vi "Main.vi"(8 "Error In":errorcluster, 10 "Output Root Directory":path=path "C:/Users/samkristoff/Desktop/dokugen output") -> (0 "Error Out":errorcluster)   [LabVIEW 2014]
panel:
  in  "Common Related Link(s)":string="[[learn:libraries:linx:reference:labview:start]] \\\\"
  in  "Relative Wiki Path":string="learn:libraries:linx:reference:labview:"
  in  "Wik Help Base URL":string="https://www.labviewmakerhub.com/doku.php?id=learn:libraries:linx:reference:labview:"
  in  "Folder Path":path=path "C:/github/makerhub/LINX/LabVIEW/vi.lib/MakerHub/LINX/Public"
  out "Progress":u8(slide)=99 scale=0.0..100.0
  out "File Path Control":path=path "C:/Program Files (x86)/National Instruments/LabVIEW 2014/vi.lib/MakerHub/LINX/Public/Utilities/Set Device User ID.vi"
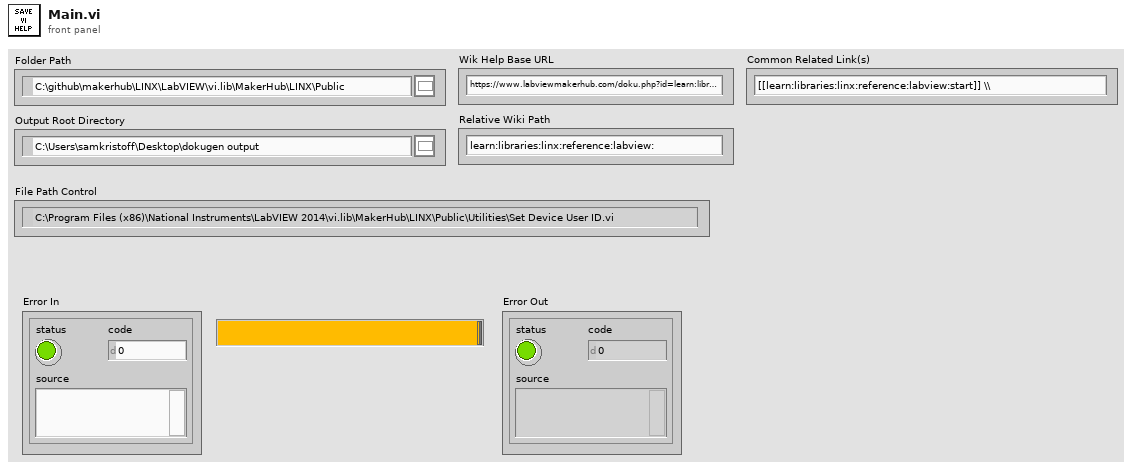
[diagram p1: front panel]
types:
  T1 = typedef "VI Data.ctl" = cluster{"Name":string, "Description":string, "Controls":T2[], "Indicators":T2[], "Connector Pane Image Data":T3, "Block Diagram Image Data":T3, "Path Tokens":string[]}
  T2 = typedef "Control Info.ctl" = cluster{"Label":string, "Description":string}
  T3 = typedef "imagedata.ctl" = cluster{"image type":i32, "image depth":i32, "image":u8[], "mask":u8[], "colors":u32[], "Rectangle":cluster{"left":i16, "top":i16, "right":i16, "bottom":i16}}
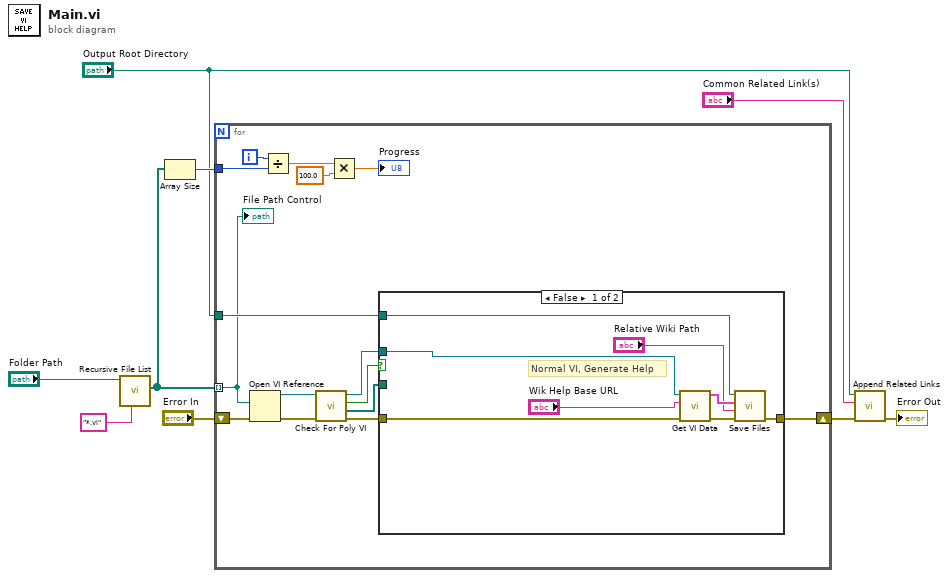
[diagram p0: block diagram]
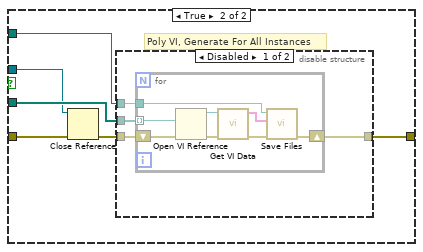
[diagram p2: hidden frame]
diagram:
  n1 = call <vilib>:"Recursive File List.vi"("pattern"="*.vi", "Folder Path"="Folder Path") -> ("All Files in Dir"=w6:path[])  [unwired: 5 in, 4 out]
  n2 = Array Size(array=w6) -> (size(s)=w5:i32)
  n3 = for {
    tunnel: "Output Root Directory" -> [w21]
    shift-right: [w20] -> w2
    shift-left: "Error In" -> [w17]
    tunnel: w6 -> [w16] mode=indexing
    tunnel: w5 -> [w13]
    i -> [w14]
    n4 = Open VI Reference(vi path=w16, error in (no error)=w17) -> (vi reference=w15:refnum<vi>, error out=w18:errorcluster)  [unwired: 4 in]
    n5 = Divide(x=w14, y=w13) -> (x/y=w12:dbl)
    n6 = call "Check For Poly VI.vi"("Error In"=w18, "VI Reference"=w15) -> ("Error Out"=w22:errorcluster, "Dependency Paths"=w23:path[], "Poly VI?"=w24:bool, "VI Reference"=w19:refnum<vi>)  [unwired: 6 in]
    n7 = Multiply(x=w12, y=100.0) -> (x*y=→"Progress":dbl)
    n8 = case shown="False" w24 {
      tunnel: w23 -> [_ w38]
      tunnel: w22 -> [w31 w34]
      tunnel: w21 -> [w26 w37]
      tunnel: [w25 w36] -> w20
      tunnel: w19 -> [w30 w35]
      frame False {
        # "Normal VI, Generate Help"
        n9 = call "Get VI Data.vi"("Error In"=w31, "Wik Help Base URL"="Wik Help Base URL", "VI Reference"=w30) -> ("Error Out"=w32:errorcluster, "VI Data"=w29:T1)  [unwired: 7 in]
        n10 = call "Save Files.vi"("Error In"=w32, "Relative Wiki Path"="Relative Wiki Path", "VI Data"=w29, "Output Root Directory"=w26) -> ("Error Out"=w25:errorcluster)  [unwired: 7 in]
      }
      frame True {
        # "Poly VI, Generate For All Instances"
        n11 = Close Reference(reference=w35, error in (no error)=w34) -> (error out=w33:errorcluster)
        n12 = disable-structure shown="Disabled" {
          disable-tunnel: w38 -> [w42 _]
          disable-tunnel: w37 -> [w41 _]
          disable-tunnel: [w40 w51] -> w36
          disable-tunnel: w33 -> [w39 w51]
          frame Disabled {
            n13 = for {
              tunnel: w42 -> [w46] mode=indexing
              shift-right: [w43] -> w40
              shift-left: w39 -> [w47]
              tunnel: w41 -> [w44]
              n14 = Open VI Reference(vi path=w46, error in (no error)=w47) -> (vi reference=w45:refnum<vi>, error out=w48:errorcluster)  [unwired: 4 in]
              n15 = call "Get VI Data.vi"("Error In"=w48, "VI Reference"=w45) -> ("Error Out"=w50:errorcluster, "VI Data"=w49:T1)  [unwired: 8 in]
              n16 = call "Save Files.vi"("Error In"=w50, "VI Data"=w49, "Output Root Directory"=w44) -> ("Error Out"=w43:errorcluster)  [unwired: 8 in]
            }
          }
          frame Enabled {
          }
        }
      }
    }
    "File Path Control" <- w16
  }
  n17 = call "Append Related Links.vi"("Error In"=w2, "Common Related Link(s)"="Common Related Link(s)", "Output Root Directory"="Output Root Directory") -> ("Error Out"=→"Error Out":errorcluster)  [unwired: 8 in]
